vi "Configure Date Format.vi"(0 "VISA resource name":refnum<visa-resource-name>, 5 "Date Format (0: Year Month Day)":u16(ring) items=["Year Month Day", "Month Day Year", "Day Month Year"], 7 "Delimiter (0: Slash(/))":u16(ring) items=["Slash (/)", "Point (.)", "Hyphen (-)"], 9 "Month Display (0: Numerical)":u16(ring) items=["Numerical", "Characters"], 11 "error in (no error)":errorcluster) -> (4 "VISA resource name out":refnum<visa-resource-name>, 15 "error out":errorcluster)   [LabVIEW 2020, in "Yokogawa GX Series.lvlib"]
doc: "Sets the date format.\n\nCommand: SDateFormat"
uses:
  <instrlib>/Yokogawa GX Series/Yokogawa GX Series.lvlib
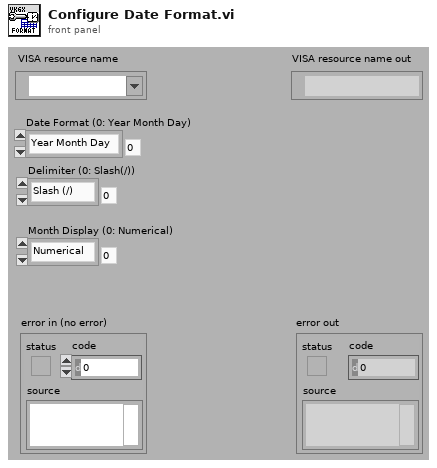
[diagram p1: front panel]
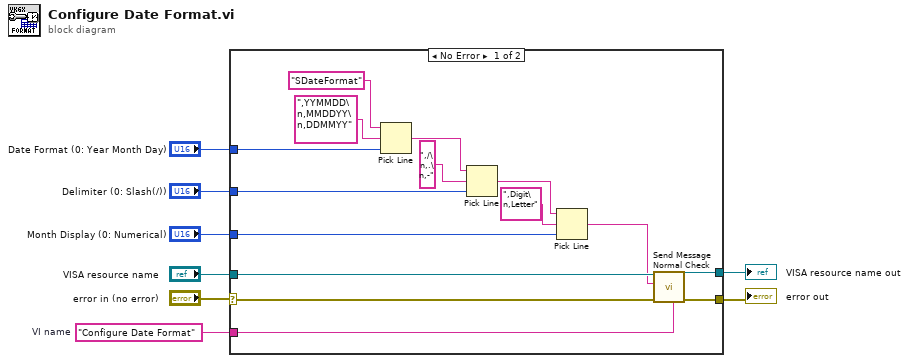
[diagram p0: block diagram]
diagram:
  w7 = "Configure Date Format"  # VI name
  n1 = case shown="No Error" "error in (no error)" {
    selector: "error in (no error)" -> [w9 w24]
    tunnel: "VISA resource name" -> [w23 w25]
    tunnel: w7 -> [w22 _]
    tunnel: [w21 w25] -> w6
    tunnel: [w20 w24] -> w5
    tunnel: "Date Format (0: Year Month Day)" -> [w17 _]
    tunnel: "Delimiter (0: Slash(/))" -> [w14 _]
    tunnel: "Month Display (0: Numerical)" -> [w10 _]
    frame No Error {
      n2 = Pick Line(string ("")="SDateFormat", multi-line string=",YYMMDD\n,MMDDYY\n,DDMMYY", line index=w17) -> (output string=w16:string)
      n3 = Pick Line(string ("")=w16, multi-line string=",/\n,.\n,-", line index=w14) -> (output string=w13:string)
      n4 = Pick Line(string ("")=w13, multi-line string=",Digit\n,Letter", line index=w10) -> (output string=w11:string)
      n5 = call <instrlib>:"Send Message Normal Check.vi"("Source (\"\")"=w22, "error in (no error)"=w9, "Send Message (\"\")"=w11, "VISA resource name"=w23) -> ("error out"=w20:errorcluster, "VISA resource name out"=w21:refnum<visa-resource-name>)  [unwired: 2 in, 4 out]
    }
    frame Error {
    }
  }
  "error out" <- w5
  "VISA resource name out" <- w6
